vi "Rotation3d_Create_RollPitchYaw.vi"(9 "Yaw":dbl, 10 "Pitch":dbl, 11 "Roll":dbl) -> (3 "Rotation3d":T1={"Q_quaternion"={"R"=1.0, "V"=[0.0, 0.0, 0.0]}})   [LabVIEW 2019, in "Trajectory_Library.lvlib"]
doc: "Constructs a Rotation3d from extrinsic roll, pitch, and yaw.\n \nExtrinsic rotations occur in that order around the axes in the fixed global frame rather than the body frame.\n \nParmeters:\n - Roll -- The counterclockwise rotation angle around the X axis (roll) in radians.\n - Pitch -- The counterclockwise rotation angle around the Y axis (pitch) in radians.\n - Yaw -- The counterclockwise rotation angle around the Z axis (yaw) in radians.\n\nReturns\n - Rotation3d -- The resulting rotation3d data cluster"
uses:
  Trajectory_Library.lvlib
  ROTATION3D.ctl
  QUATERNION.ctl
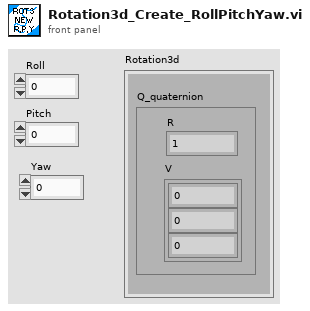
[diagram p1: front panel]
types:
  T1 = typedef "Trajectory_Library.lvlib/ROTATION3D.ctl" = cluster{"Q_quaternion":T2}
  T2 = typedef "Trajectory_Library.lvlib/QUATERNION.ctl" = cluster{"R":dbl, "V":dbl[]}
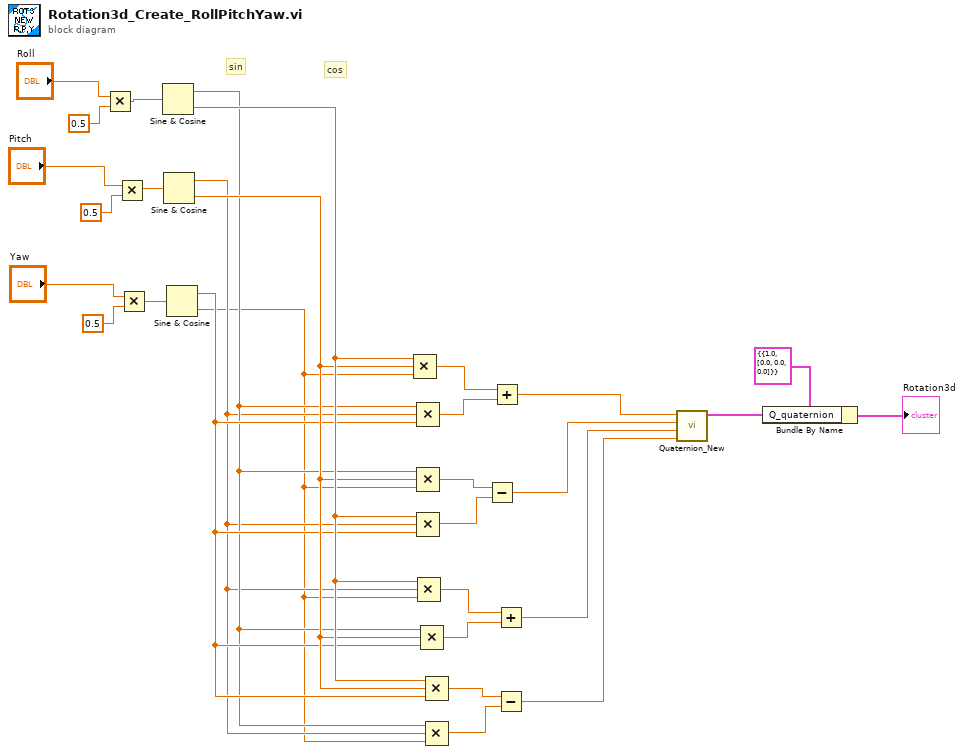
[diagram p0: block diagram]
diagram:
  # "cos"
  # "sin"
  n1 = Multiply(x="Roll", y=0.5) -> (x*y=w19:dbl)
  n2 = Multiply(x="Pitch", y=0.5) -> (x*y=w20:dbl)
  n3 = Multiply(x="Yaw", y=0.5) -> (x*y=w21:dbl)
  n4 = Sine & Cosine(0:w19) -> (1:w3:dbl, 2:w6:dbl)
  n5 = Sine & Cosine(0:w20) -> (1:w2:dbl, 2:w5:dbl)
  n6 = Sine & Cosine(0:w21) -> (1:w4:dbl, 2:w1:dbl)
  n7 = Compound Arithmetic op=MULTIPLY(w6, w5, w1) -> (w18:dbl)
  n8 = Compound Arithmetic op=MULTIPLY(w3, w2, w4) -> (w17:dbl)
  n9 = Compound Arithmetic op=MULTIPLY(w3, w5, w1) -> (w15:dbl)
  n10 = Compound Arithmetic op=MULTIPLY(w6, w2, w4) -> (w14:dbl)
  n11 = Compound Arithmetic op=MULTIPLY(w6, w2, w1) -> (w12:dbl)
  n12 = Compound Arithmetic op=MULTIPLY(w3, w5, w4) -> (w11:dbl)
  n13 = Compound Arithmetic op=MULTIPLY(w6, w5, w4) -> (w9:dbl)
  n14 = Compound Arithmetic op=MULTIPLY(w3, w2, w1) -> (w8:dbl)
  n15 = Subtract(x=w15, y=w14) -> (x-y=w13:dbl)
  n16 = Add(x=w18, y=w17) -> (x+y=w16:dbl)
  n17 = Add(x=w12, y=w11) -> (x+y=w10:dbl)
  n18 = Subtract(x=w9, y=w8) -> (x-y=w7:dbl)
  n19 = call "Quaternion_New.vi"("Z"=w7, "Y"=w10, "X"=w13, "W"=w16) -> ("out Quaternion"=w28:T2)  [unwired: 7 in]
  n20 = Bundle By Name(cluster=T1 {"Q_quaternion"={"R"=1.0, "V"=[0.0, 0.0, 0.0]}} ("ROTATION3D"), "Q_quaternion"=w28) -> (→"Rotation3d":T1)
